vi "GUI Path Locations.vi"(7 "Enum":T1=enum."Vibratome GUI", 8 "Error In":errorcluster) -> (0 "Error Out":errorcluster, 2 "file or folder exists?":bool, 3 "GUI Path":path)   [LabVIEW 2014]
uses:
  Controls/GUI Types.ctl
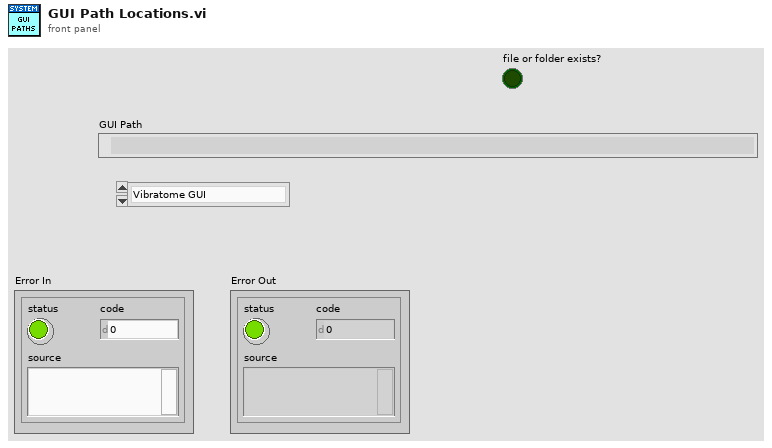
[diagram p1: front panel]
types:
  T1 = typedef "GUI Types.ctl" = enum16{"Mosaic GUI", "Vibratome GUI"}
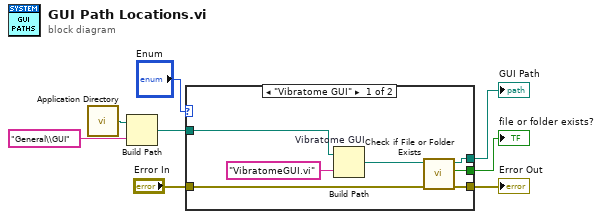
[diagram p0: block diagram]
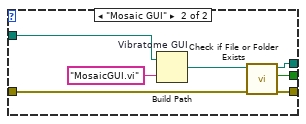
[diagram p2: hidden frame]
diagram:
  n1 = call <vilib>:"Application Directory.vi"() -> ("Application Directory"=w7:path)
  n2 = Build Path(base path=w7, name or relative path="General\\GUI") -> (appended path=w6:path)
  n3 = case shown="\"Vibratome GUI\"" "Enum" {
    tunnel: w6 -> [w13 w20]
    tunnel: [w12 w19] -> w4
    tunnel: [w11 w18] -> w3
    tunnel: [w9 w17] -> w2
    tunnel: "Error In" -> [w10 w16]
    frame "Vibratome GUI" {
      n4 = Build Path "Vibratome GUI"(base path=w13, name or relative path="VibratomeGUI.vi") -> (appended path=w15:path)
      n5 = call <vilib>:"Check if File or Folder Exists.vi"("error in (no error)"=w10, "path"=w15) -> ("error out"=w9:errorcluster, "file or folder exists?"=w11:bool, "dup path"=w12:path)  [unwired: 7 in]
    }
    frame "Mosaic GUI" {
      n6 = Build Path "Vibratome GUI"(base path=w20, name or relative path="MosaicGUI.vi") -> (appended path=w22:path)
      n7 = call <vilib>:"Check if File or Folder Exists.vi"("error in (no error)"=w16, "path"=w22) -> ("error out"=w17:errorcluster, "file or folder exists?"=w18:bool, "dup path"=w19:path)  [unwired: 7 in]
    }
  }
  "GUI Path" <- w4
  "file or folder exists?" <- w3
  "Error Out" <- w2
